vi "Pool Avg.vi"(1 "Input":dbl) -> (0 "Output Avg":dbl)   [LabVIEW 2011]
panel:
  out "Minimum":dbl
  out "Maximum":dbl
  in  "Sample Size":i32
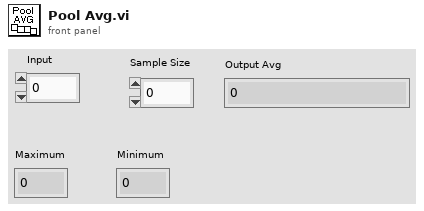
[diagram p1: front panel]
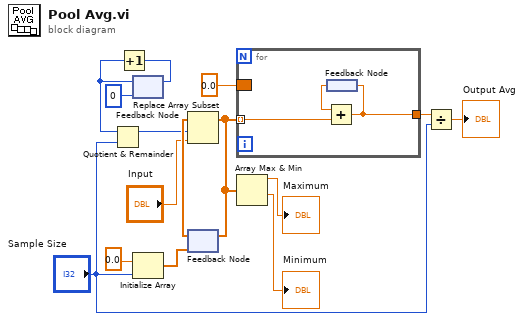
[diagram p0: block diagram]
diagram:
  n1 = feedback #1(0) -> (w9:i32)
  n2 = Quotient & Remainder(x=w9, y="Sample Size") -> (x-y*floor(x/y)=w8:i32)  [unwired: 1 out]
  n3 = Increment(x=w9) -> (x+1=w10:i32)
  n4 = feedback-in #1(w10) -> ()
  n5 = Initialize Array(0.0 ("element"), "Sample Size") -> (w14:dbl[])
  n6 = feedback #2(w14) -> (w13:dbl[])
  n7 = Replace Array Subset(array=w13, new element="Input", index=w8) -> (w3:dbl[])
  n8 = feedback-in #2(w3) -> ()
  n9 = for {
    tunnel: w3 -> [w17] mode=indexing
    tunnel: [w16] -> w7
    border: 0.0 -> [_]
    n10 = feedback #3() -> (w18:dbl)
    n11 = Add(x=w18, y=w17) -> (x+y=w16:dbl)
    n12 = feedback-in #3(w16) -> ()
  }
  n13 = Array Max & Min(array=w3) -> (max value=→"Maximum":dbl, min value=→"Minimum":dbl)  [unwired: 2 out]
  n14 = Divide(x=w7, y="Sample Size") -> (x/y=→"Output Avg":dbl)
